vi "Size.vi"(8 "error in (no error)":errorcluster, 11 "Data Class Array in":refnum<class "Data Class Array.lvclass">) -> (0 "error out":errorcluster, 2 "Size":i32, 3 "Data Class Array out":refnum<class "Data Class Array.lvclass">)   [LabVIEW 2020, in "Data.lvlib" / "Data Class Array.lvclass"]
doc: "Return the size of the generic data element."
uses:
  Data Class Array.lvclass
  Data Class Array.lvclass/Data Class Array.ctl
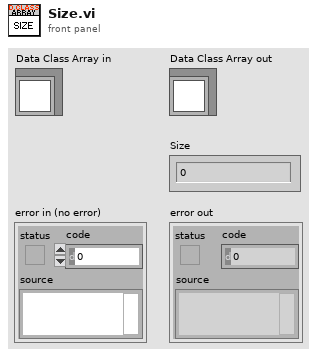
[diagram p1: front panel]
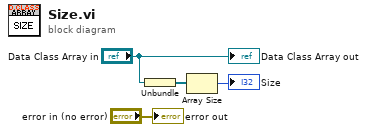
[diagram p0: block diagram]
diagram:
  n1 = Unbundle("Data Class Array in") -> (w2:refnum<class "Data Class.lvclass">[])
  n2 = Array Size(array=w2) -> (size(s)=→"Size":i32)
  "error out" <- "error in (no error)"
  "Data Class Array out" <- "Data Class Array in"
